vi "ISOOCV.vi"() -> ()   [LabVIEW 2020]
panel:
  in  "ISO OCV":string
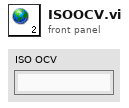
[diagram p1: front panel]
diagram:
